vi "WPI_DriverStationCreate Lib Version File.vi"(8 "error in":errorcluster) -> (0 "error out":errorcluster)   [LabVIEW 2017]
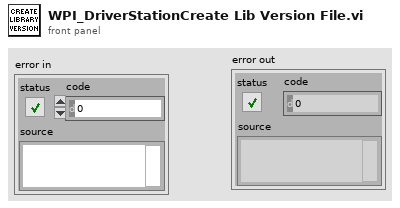
[diagram p1: front panel]
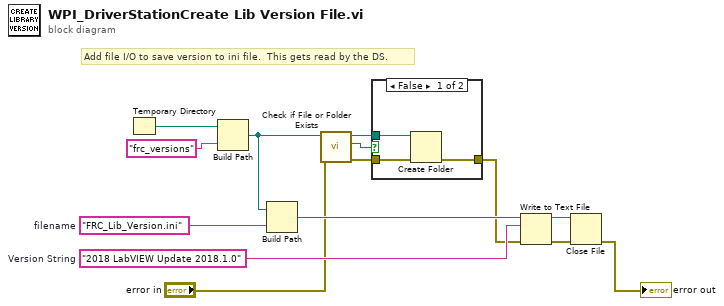
[diagram p0: block diagram]
diagram:
  w11 = "FRC_Lib_Version.ini"  # filename
  w13 = "2018 LabVIEW Update 2018.1.0"  # Version String
  # "Add file I/O to save version to ini file.  This gets read by the DS."
  n1 = Temporary Directory() -> (w10:path)
  n2 = Build Path(base path=w10, name or relative path="frc_versions") -> (appended path=w5:path)
  n3 = Build Path(base path=w5, name or relative path=w11) -> (appended path=w12:path)
  n4 = call <vilib>:"Check if File or Folder Exists.vi"("error in (no error)"="error in", "path"=w5) -> ("error out"=w1:errorcluster, "file or folder exists?"=w3:bool, "dup path"=w4:path)  [unwired: 7 in]
  n5 = case shown="False" w3 {
    tunnel: [w17 w18] -> w8
    tunnel: w4 -> [w16 _]
    tunnel: w1 -> [w15 w18]
    frame False {
      n6 = Create Folder(path (use dialog)=w16, error in=w15) -> (error out=w17:errorcluster)  [unwired: 1 in, 2 out]
    }
    frame True {
      # "don't create if folder already exists"
    }
  }
  n7 = Write to Text File(file (use dialog)=w12, text=w13, error in=w8) -> (refnum out=w14:refnum<file>, error out=w7:errorcluster)  [unwired: 1 in, 1 out]
  n8 = Close File(refnum=w14, error in=w7) -> (error out=→"error out":errorcluster)  [unwired: 1 out]
